vi "Simulate Self Test.vi"(8 "error in (no error)":errorcluster, 11 "Device Under Test In":refnum<class "Device Under Test.lvclass">) -> (0 "error out":errorcluster, 2 "Pass":bool, 3 "Device Under Test Out":refnum<class "Device Under Test.lvclass">)   [LabVIEW 2020, in "Device Under Test.lvclass"]
uses:
  Device Under Test.lvclass
  Device Under Test.lvclass/Device Under Test.ctl
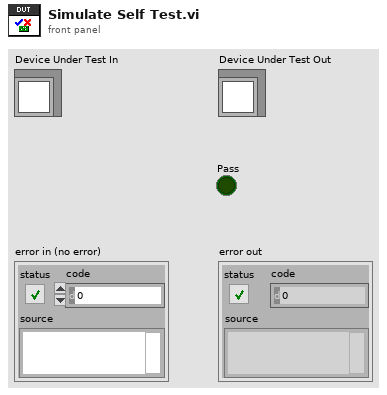
[diagram p1: front panel]
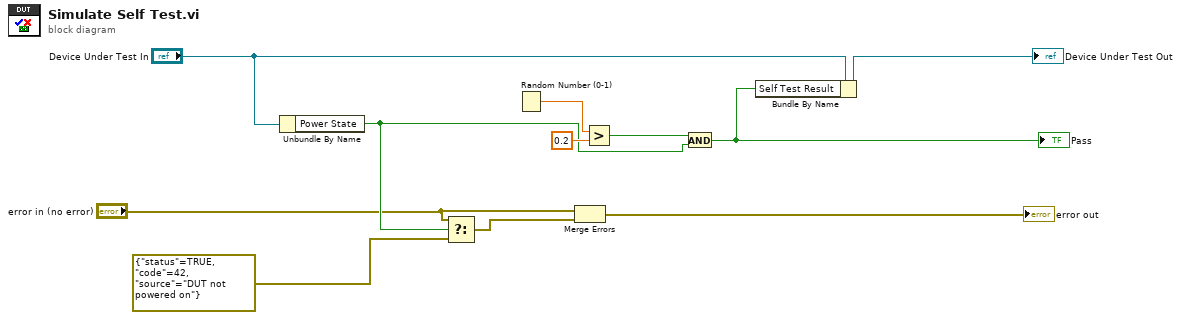
[diagram p0: block diagram]
diagram:
  n1 = Unbundle By Name("Device Under Test In") -> ("Power State"=w7:bool)
  n2 = Select(t="error in (no error)", s=w7, f=errorcluster {"status"=TRUE, "code"=42, "source"="DUT not powered on"}) -> (s? t:f=w6:errorcluster)
  n3 = Random Number (0-1)() -> (number: 0 to 1=w11:dbl)
  n4 = Merge Errors("error in (no error)", w6) -> (→"error out":errorcluster)
  n5 = Greater?(x=w11, y=0.2) -> (0:w9:bool)
  n6 = And(x=w9, y=w7) -> (x .and. y?=w1:bool)
  "Pass" <- w1
  n7 = Bundle By Name(cluster="Device Under Test In", "Self Test Result"=w1) -> (→"Device Under Test Out":refnum<class "Device Under Test.lvclass">)
